vi "Agilent Oscilloscope run and stop.vi"() -> ()   [LabVIEW 2011]
uses:
  <vilib>/Instr/_visa.llb/VISA Open Access Mode.ctl
panel:
  in  "run time (ms)":u32=1000
  out "error out":errorcluster
  in  "VISA GPIB Resource":refnum<visa-resource-name>="GPIB0::7::INSTR"
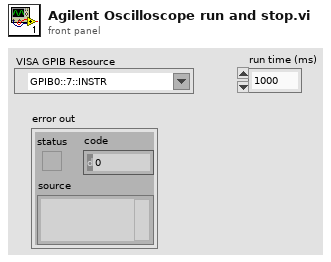
[diagram p1: front panel]
types:
  T1 = typedef "VISA Open Access Mode.ctl" = u32
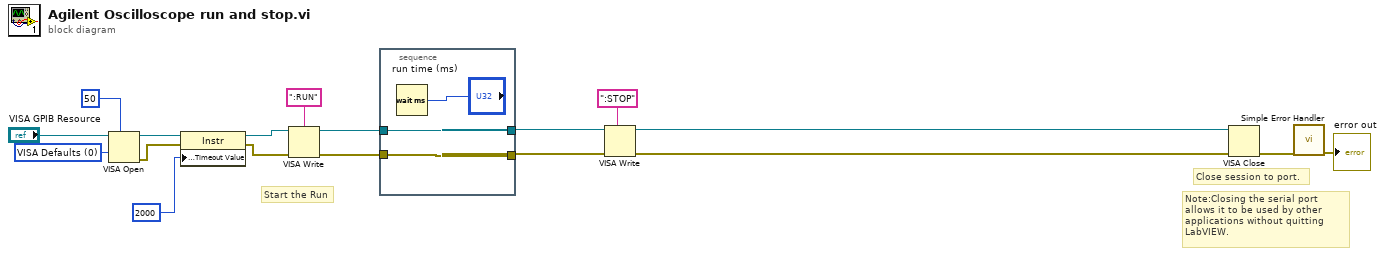
[diagram p0: block diagram]
diagram:
  w11 = T1 0 items=["VISA Defaults"=0, "Exclusive Lock"=1, "Load Configured Settings"=4] ("Access Mode")
  # "Start the Run"
  # "Note:Closing the serial port allows it to be used by other applications without quitting LabVIEW."
  # "Close session to port."
  n1 = VISA Open(timeout (0)=u32 50 ("VISA Open timeout (0)"), access mode=w11, VISA resource name="VISA GPIB Resource") -> (VISA resource name=w14:refnum<visa-resource-name>, error out=w13:errorcluster)  [unwired: 2 in]
  n2 = property class="Instr"(reference=w14, error in=w13, "General Settings:Timeout Value"=u32 2000) -> (reference out=w10:refnum<visa-resource-name>, error out=w9:errorcluster)
  n3 = VISA Write(VISA resource name=w10, write buffer=":RUN" ("string to write"), error in (no error)=w9) -> (VISA resource name out=w4:refnum<visa-resource-name>, error out=w2:errorcluster)  [unwired: 1 out]
  n4 = stacked-sequence {
    tunnel: w4 -> [w20]
    tunnel: [w20] -> w3
    tunnel: w2 -> [w19]
    tunnel: [w19] -> w1
    frame #0 {
      n5 = Wait (ms)(milliseconds to wait="run time (ms)") -> ()  [unwired: 1 out]
    }
  }
  n6 = VISA Write(VISA resource name=w3, write buffer=":STOP" ("string to write"), error in (no error)=w1) -> (VISA resource name out=w5:refnum<visa-resource-name>, error out=w6:errorcluster)  [unwired: 1 out]
  n7 = VISA Close(VISA resource name=w5, error in (no error)=w6) -> (error out=w18:errorcluster)
  n8 = call <vilib>:"Simple Error Handler.vi"("error in (no error)"=w18) -> ("error out"=→"error out":errorcluster)  [unwired: 1 in, 7 out]
